vi "Untitled 2.vi"() -> ()   [LabVIEW 2017]
panel:
  in  "stop":bool
  in  "DIO0":bool
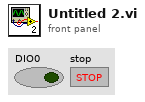
[diagram p1: front panel]
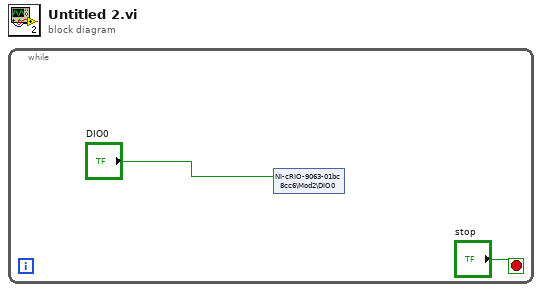
[diagram p0: block diagram]
diagram:
  n1 = while {
    stop <- "stop" stop-if-true
    n2 = shared-variable "NI-cRIO-9063-01bc8cc6\\Mod2\\DIO0"("DIO0") -> ()  [unwired: 1 in, 1 out]
  }
